vi "Example - DataType Timestamp.vi"() -> ()   [LabVIEW 2017]
uses:
  API-String-Arugments-Support/API String Arguments Support.lvlib
panel:
  in  "Empty String":string
  out "error 4":errorcluster
  out "data 4":timestamp=timestamp(3781608579.597 s since 1904-01-01)
  in  "UTC? (F)":bool=TRUE
  out "String 4":string="2023-10-31T14:49:39.597Z"
  in  "Time Stamp 4":timestamp=timestamp(3781608579.597416 s since 1904-01-01)
  out "Timestamp 4'":timestamp
  out "String 3":string="2023-10-31T14:49:39.597Z"
  out "data 3":timestamp=timestamp(3779880873 s since 1904-01-01)
  out "data 2":timestamp=timestamp(3781608579.597 s since 1904-01-01)
  out "Timestamp 1'":timestamp=timestamp(3781608579.597 s since 1904-01-01)
  out "concatenated string":string="2023-10-11 22:54:33(%<%Y-%m-%d %H:%M:%S>T)"
  out "error 3":errorcluster
  out "error 2":errorcluster
  in  "String 2":string="2023-10-31T14:49:39.597Z"
  in  "Time Stamp 3":timestamp=timestamp(3779880873.3011937 s since 1904-01-01)
  out "error":errorcluster
  in  "Time Stamp 1":timestamp=timestamp(3781608579.597416 s since 1904-01-01)
  out "String":string="2023-10-31T14:49:39.597Z"
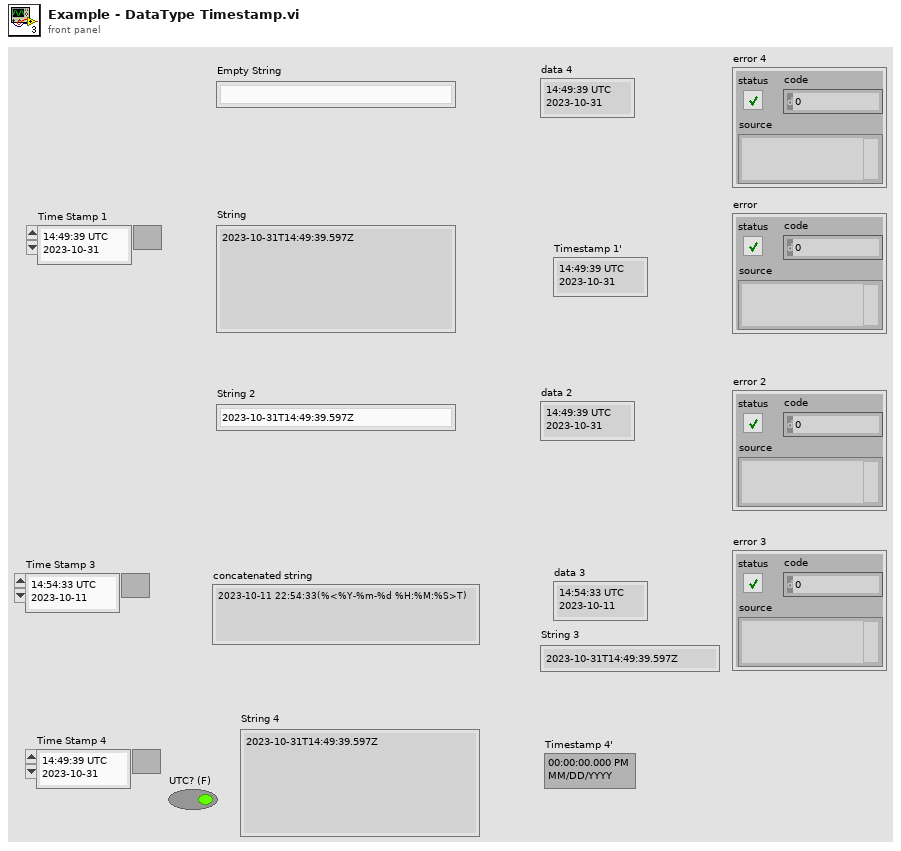
[diagram p1: front panel]
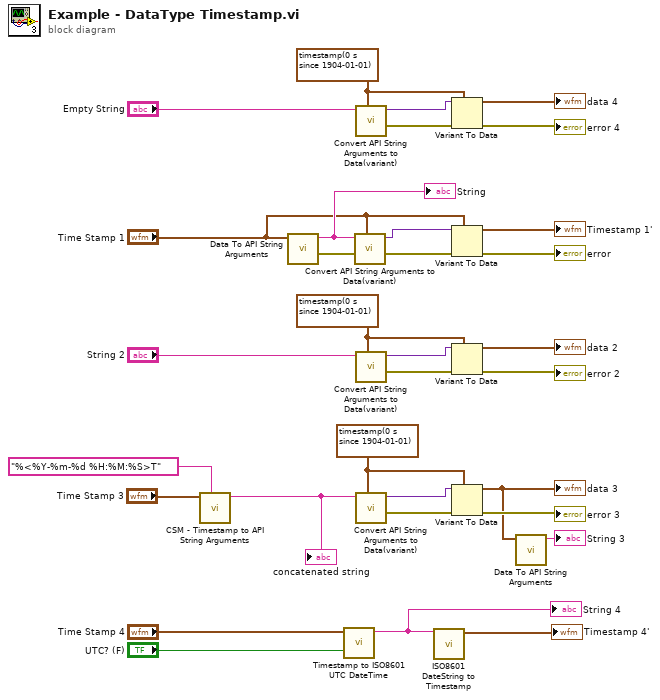
[diagram p0: block diagram]
diagram:
  w5 = timestamp(0 s since 1904-01-01) ("Time Stamp")
  w23 = timestamp(0 s since 1904-01-01) ("Time Stamp")
  w20 = timestamp(0 s since 1904-01-01) ("Time Stamp")
  n1 = call "CSM - Timestamp to API String Arguments.vi"("Format(Empty to use UTC)"="%<%Y-%m-%d %H:%M:%S>T" ("format string"), "Timestamp (now)"="Time Stamp 3") -> ("CSM Timestamp Argument"=w7:string)  [unwired: 9 in]
  "concatenated string" <- w7
  n2 = call "Data To API String Arguments.vi"("data"="Time Stamp 1") -> ("error out"=w31:errorcluster, "String"=w32:string)  [unwired: 9 in]
  "String" <- w32
  n3 = call <vilib>:"Timestamp to ISO8601 UTC DateTime.vi"("UTC? (F)"="UTC? (F)", "Timestamp (now)"="Time Stamp 4") -> ("ISO8601 String"=w11:string)  [unwired: 9 in]
  "String 4" <- w11
  n4 = call "Convert API String Arguments to Data(variant).vi"("Type"="Time Stamp 1", "error in (no error)"=w31, "String"=w32) -> ("error"=w30:errorcluster, "Data"=w18:variant)  [unwired: 7 in]
  n5 = call "Convert API String Arguments to Data(variant).vi"("Type"=w5, "String"="Empty String") -> ("error"=w2:errorcluster, "Data"=w4:variant)  [unwired: 8 in]
  n6 = call "Convert API String Arguments to Data(variant).vi"("Type"=w20, "String"="String 2") -> ("error"=w28:errorcluster, "Data"=w21:variant)  [unwired: 8 in]
  n7 = call "Convert API String Arguments to Data(variant).vi"("Type"=w23, "String"=w7) -> ("error"=w27:errorcluster, "Data"=w22:variant)  [unwired: 8 in]
  n8 = call <vilib>:"ISO8601 DateString to Timestamp.vi"("ISO8601 String"=w11) -> ("Timestamp"=→"Timestamp 4'":timestamp)  [unwired: 8 in, 2 out]
  n9 = Variant To Data(error in=w2, type=w5, Variant=w4) -> (data=→"data 4":timestamp, error out=→"error 4":errorcluster)
  n10 = Variant To Data(error in=w30, type="Time Stamp 1", Variant=w18) -> (data=→"Timestamp 1'":timestamp, error out=→"error":errorcluster)
  n11 = Variant To Data(error in=w28, type=w20, Variant=w21) -> (data=→"data 2":timestamp, error out=→"error 2":errorcluster)
  n12 = Variant To Data(error in=w27, type=w23, Variant=w22) -> (data=w15:timestamp, error out=→"error 3":errorcluster)
  "data 3" <- w15
  n13 = call "Data To API String Arguments.vi"("data"=w15) -> ("String"=→"String 3":string)  [unwired: 9 in, 1 out]
